vi "open connection.vi"(8 "error in (no error)":errorcluster caption="Fehler (Eingang, kein Fehler)", 11 "Class 4 Eingang":refnum<class "Class 4.lvclass"> caption="DNL_LabVIEW Object in") -> (0 "error out":errorcluster caption="Fehler (Ausgang)", 3 "Class 4 Ausgang":refnum<class "Class 4.lvclass"> caption="DNL_LabVIEW Object out")   [LabVIEW 2013, in "Class 4.lvclass"]
doc: "Verbindung zu dem Gerät öffnen"
uses:
  Class 4.lvclass
  DeviceInterface/DeviceInterface.lvclass
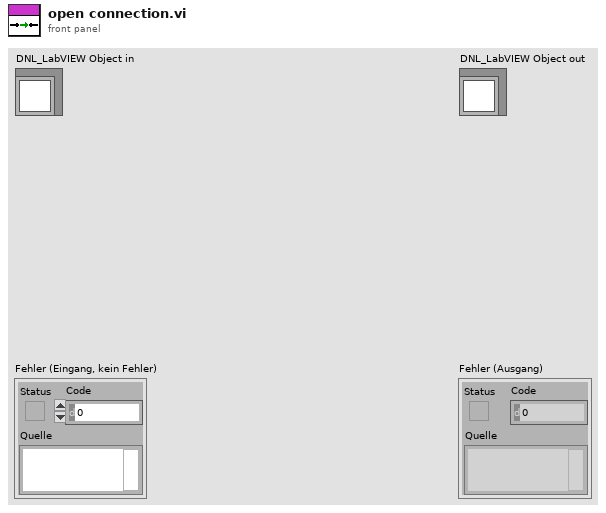
[diagram p1: front panel]
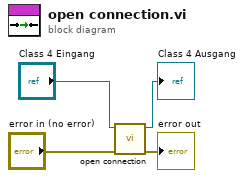
[diagram p0: block diagram]
diagram:
  n1 = call-parent "open connection.vi"("error in (no error)"="error in (no error)", "DeviceInterface Eingang"="Class 4 Eingang") -> ("error out"=→"error out":errorcluster, "DeviceInterface Ausgang"=→"Class 4 Ausgang":refnum<class "Class 4.lvclass">)  [unwired: 8 in]
